vi "LS330_RampGo.vi"(5 "Ramp Rate":dbl, 6 "Final Temp (K)":dbl, 7 "Initial Temp (K)":dbl, 8 "error in":errorcluster, 9 "Range":T1, 10 "Heater":string(combo)="1", 11 "VISA resource name":refnum<visa-resource-name>) -> (0 "error out":errorcluster, 3 "VISA resource name out":refnum<visa-resource-name>)   [LabVIEW 2021]
uses:
  Heater_Range.ctl
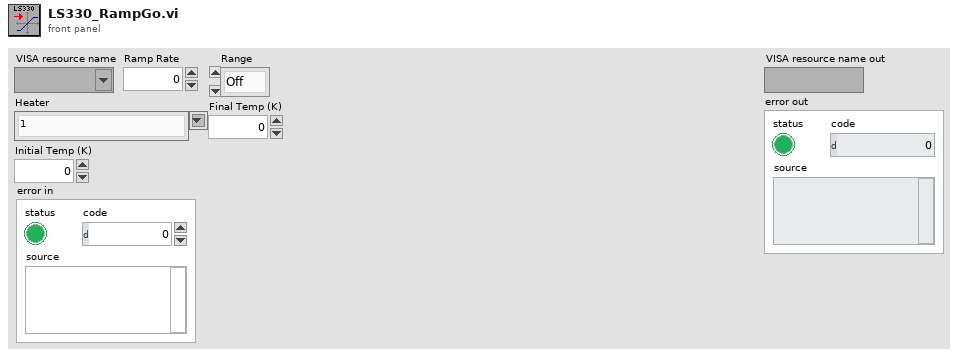
[diagram p1: front panel]
types:
  T1 = typedef "Heater_Range.ctl" = enum16{"Off", "Low", "Medium", "High"}
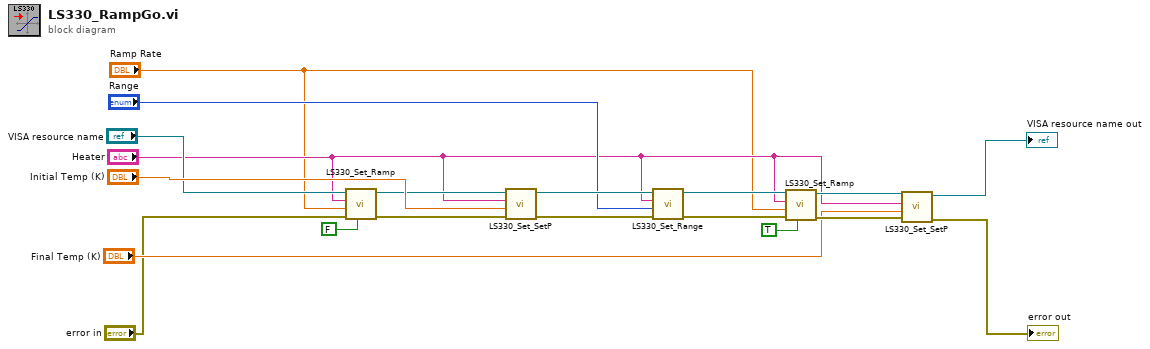
[diagram p0: block diagram]
diagram:
  n1 = call "LS330_Set_Ramp.vi"("Ramp Toggle"=FALSE, "error in"="error in", "Ramp Rate"="Ramp Rate", "Heater"="Heater", "VISA resource name"="VISA resource name") -> ("error out"=w7:errorcluster, "VISA resource name out"=w5:refnum<visa-resource-name>)  [unwired: 4 in]
  n2 = call "LS330_Set_SetP.vi"("error in"=w7, "Set Temp (K)"="Initial Temp (K)", "Heater"="Heater", "VISA resource name"=w5) -> ("error out"=w17:errorcluster, "VISA resource name out"=w18:refnum<visa-resource-name>)  [unwired: 5 in]
  n3 = call "LS330_Set_Range.vi"("error in"=w17, "Range"="Range", "Heater"="Heater", "VISA resource name"=w18) -> ("error out"=w14:errorcluster, "VISA resource name out"=w15:refnum<visa-resource-name>)  [unwired: 5 in]
  n4 = call "LS330_Set_Ramp.vi"("Ramp Toggle"=TRUE, "error in"=w14, "Ramp Rate"="Ramp Rate", "Heater"="Heater", "VISA resource name"=w15) -> ("error out"=w12:errorcluster, "VISA resource name out"=w13:refnum<visa-resource-name>)  [unwired: 4 in]
  n5 = call "LS330_Set_SetP.vi"("error in"=w12, "Set Temp (K)"="Final Temp (K)", "Heater"="Heater", "VISA resource name"=w13) -> ("error out"=→"error out":errorcluster, "VISA resource name out"=→"VISA resource name out":refnum<visa-resource-name>)  [unwired: 5 in]
